vi "getSpecStatus.vi"(8 "error in":T1, 11 "index":i32) -> (0 "error out":T1, 3 "specstatus":i32)   [LabVIEW 2016]
doc: "Returns the current status of the spectroscopy engine. Differentiated is specstatus = 0 if the engine does not run and specstatus = 1 if the engine runs.\nWith the index-input you can define which spec-engine you want to know the status from (index 0-2 corresponds to the engines 1-3)."
uses:
  Controls/Error_Out.ctl
  Files_ASC500/DLL/ASC500_RemoteControlV27.dll
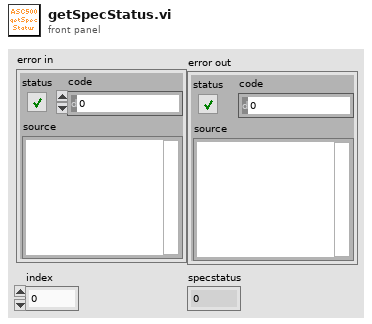
[diagram p1: front panel]
types:
  T1 = typedef "Error_Out.ctl" = errorcluster
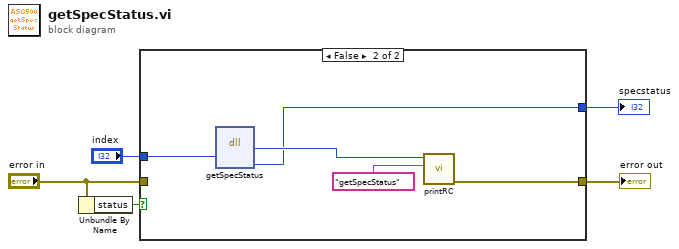
[diagram p0: block diagram]
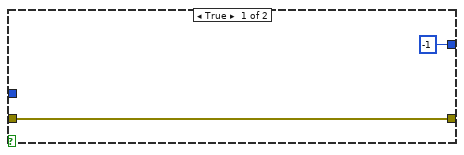
[diagram p2: hidden frame]
diagram:
  n1 = Unbundle By Name("error in") -> ("status"=w5:bool)
  n2 = case shown="False" w5 {
    tunnel: "error in" -> [w7 _]
    tunnel: [w7 w12] -> w3
    tunnel: "index" -> [_ w9]
    tunnel: [-1 ("Status") w8] -> w1
    frame True {
    }
    frame False {
      n3 = dll-call lib="G:/SCMOperations/Share/ELE/Produkt Information/ASC500/04 Remote Control/02 development versions/2018Nov06/Files_ASC500/DLL/ASC500_RemoteControlV27.dll" fn="getSpecStatus"("index"=w9) -> ("return type"=w11:i32, "specstatus"=w8:i32)  [unwired: 5 in, 2 out]
      n4 = call "printRC.vi"("additional information"="getSpecStatus", "RC"=w11) -> ("error out"=w12:T1)  [unwired: 9 in]
    }
  }
  "error out" <- w3
  "specstatus" <- w1
